vi "Test XML Objects.vi"() -> ()   [LabVIEW 2013]
uses:
  Shifter.lvclass
  Shifters.lvclass
  ACNET Device Limits List.lvclass
  ACNET Device Limits.lvclass
panel:
  out "Device Limits":string
  out "Device Range States":cluster{"name":string, dbl, "Numeric":i8}[](array[cluster]) {"?" format="%_6g"}
  out "Shifter List XML":string
  out "Shifter XML":string
  out "phoneNumbers":string[](array[string])
  out "emails":string[](array[string])
  out "name":string
  in  "XML File Path":path=path "C:/Users/plane/Dropbox/Research/MTA/DAQ VIs/XML Objects/Test Shifter Object.xml"
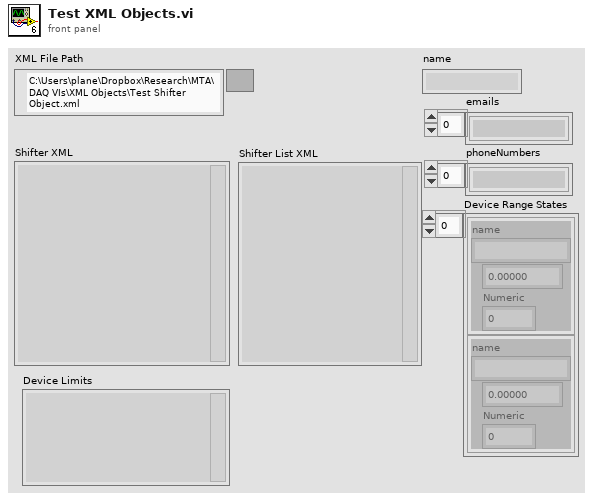
[diagram p1: front panel]
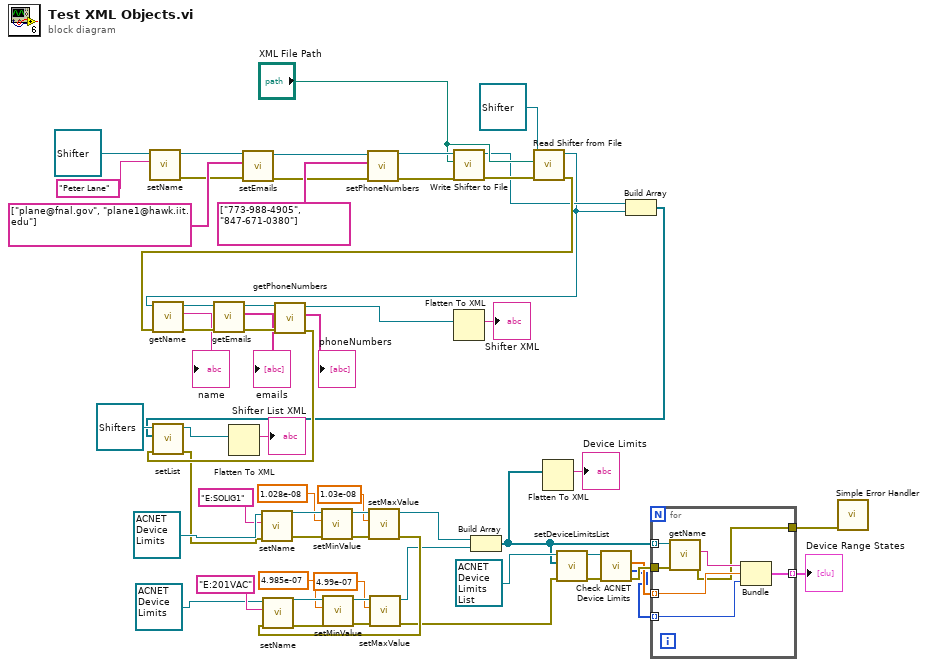
[diagram p0: block diagram]
diagram:
  n1 = call-dynamic "setName.vi"("name"="Peter Lane", "Shifter in"=refnum<class "Shifter.lvclass"> refnum ("Shifter.lvclass")) -> ("error out"=w54:errorcluster, "Shifter out"=w59:refnum<class "Shifter.lvclass">)  [unwired: 8 in]
  n2 = call-dynamic "setEmails.vi"("error in (no error)"=w54, "emails"=string[] ["plane@fnal.gov", "plane1@hawk.iit.edu"], "Shifter in"=w59) -> ("error out"=w53:errorcluster, "Shifter out"=w56:refnum<class "Shifter.lvclass">)  [unwired: 7 in]
  n3 = call-dynamic "setPhoneNumbers.vi"("error in (no error)"=w53, "phoneNumbers"=string[] ["773-988-4905", "847-671-0380"], "Shifter in"=w56) -> ("error out"=w52:errorcluster, "Shifter out"=w55:refnum<class "Shifter.lvclass">)  [unwired: 7 in]
  n4 = call "Write Shifter to File.vi"("error in (no error)"=w52, "XML File Path"="XML File Path", "Shifter in"=w55) -> ("error out"=w51:errorcluster, "Shifter out"=w36:refnum<class "Shifter.lvclass">)  [unwired: 7 in]
  n5 = call "Read Shifter from File.vi"("error in (no error)"=w51, "XML File Path"="XML File Path", "Shifter in"=refnum<class "Shifter.lvclass"> refnum) -> ("error out"=w48:errorcluster, "Shifter out"=w35:refnum<class "Shifter.lvclass">)  [unwired: 7 in]
  n6 = call-dynamic "getName.vi"("error in (no error)"=w48, "Shifter in"=w35) -> ("error out"=w45:errorcluster, "name"=→"name":string, "Shifter out"=w47:refnum<class "Shifter.lvclass">)  [unwired: 7 in]
  n7 = call-dynamic "getEmails.vi"("error in (no error)"=w45, "Shifter in"=w47) -> ("error out"=w44:errorcluster, "emails"=→"emails":string[], "Shifter out"=w46:refnum<class "Shifter.lvclass">)  [unwired: 7 in]
  n8 = call-dynamic "getPhoneNumbers.vi"("error in (no error)"=w44, "Shifter in"=w46) -> ("error out"=w37:errorcluster, "phoneNumbers"=→"phoneNumbers":string[], "Shifter out"=w39:refnum<class "Shifter.lvclass">)  [unwired: 7 in]
  n9 = Flatten To XML(anything=w39) -> (xml string=→"Shifter XML":string)
  n10 = Build Array(w36, w35) -> (w34:refnum<class "Shifter.lvclass">[])
  n11 = call-dynamic "setList.vi"("error in (no error)"=w37, "list"=w34, "Shifters in"=refnum<class "Shifters.lvclass"> refnum) -> ("error out"=w29:errorcluster, "Shifters out"=w33:refnum<class "Shifters.lvclass">)  [unwired: 7 in]
  n12 = Flatten To XML(anything=w33) -> (xml string=→"Shifter List XML":string)
  n13 = call-dynamic "setName.vi"("error in (no error)"=w29, "name"="E:SOLIG1", "ACNET Device Limits in"=refnum<class "ACNET Device Limits.lvclass"> refnum ("ACNET Device Limits.lvclass")) -> ("error out"=w27:errorcluster, "ACNET Device Limits out"=w28:refnum<class "ACNET Device Limits.lvclass">)  [unwired: 7 in]
  n14 = call-dynamic "setMinValue.vi"("error in (no error)"=w27, "minValue"=1.028e-08, "ACNET Device Limits in"=w28) -> ("error out"=w24:errorcluster, "ACNET Device Limits out"=w25:refnum<class "ACNET Device Limits.lvclass">)  [unwired: 7 in]
  n15 = call-dynamic "setMaxValue.vi"("error in (no error)"=w24, "maxValue"=1.03e-08, "ACNET Device Limits in"=w25) -> ("error out"=w17:errorcluster, "ACNET Device Limits out"=w13:refnum<class "ACNET Device Limits.lvclass">)  [unwired: 7 in]
  n16 = call-dynamic "setName.vi"("error in (no error)"=w17, "name"="E:201VAC", "ACNET Device Limits in"=refnum<class "ACNET Device Limits.lvclass"> refnum ("ACNET Device Limits.lvclass")) -> ("error out"=w15:errorcluster, "ACNET Device Limits out"=w21:refnum<class "ACNET Device Limits.lvclass">)  [unwired: 7 in]
  n17 = call-dynamic "setMinValue.vi"("error in (no error)"=w15, "minValue"=4.985e-07, "ACNET Device Limits in"=w21) -> ("error out"=w14:errorcluster, "ACNET Device Limits out"=w19:refnum<class "ACNET Device Limits.lvclass">)  [unwired: 7 in]
  n18 = call-dynamic "setMaxValue.vi"("error in (no error)"=w14, "maxValue"=4.99e-07, "ACNET Device Limits in"=w19) -> ("error out"=w10:errorcluster, "ACNET Device Limits out"=w12:refnum<class "ACNET Device Limits.lvclass">)  [unwired: 7 in]
  n19 = Build Array(w13, w12) -> (w3:refnum<class "ACNET Device Limits.lvclass">[])
  n20 = Flatten To XML(anything=w3) -> (xml string=→"Device Limits":string)
  n21 = call-dynamic "setDeviceLimitsList.vi"("error in (no error)"=w10, "Device Limits List"=w3, "ACNET Device Checker in"=refnum<class "ACNET Device Limits List.lvclass"> refnum ("ACNET Device Checker.lvclass")) -> ("error out"=w9:errorcluster, "ACNET Device Checker out"=w8:refnum<class "ACNET Device Limits List.lvclass">)  [unwired: 7 in]
  n22 = call "Check ACNET Device Limits.vi"("error in (no error)"=w9, "ACNET Device Limits List in"=w8) -> ("error out"=w7:errorcluster, "Range States"=w5:i8[], "Values"=w6:dbl[])  [unwired: 6 in, 1 out]
  n23 = for {
    tunnel: w3 -> [w68] mode=indexing
    tunnel: w7 -> [w67]
    tunnel: w6 -> [w65] mode=indexing
    tunnel: w5 -> [w64] mode=indexing
    tunnel: [w63] -> w4 mode=indexing
    tunnel: [w62] -> w1
    n24 = call-dynamic "getName.vi"("error in (no error)"=w67, "ACNET Device Limits in"=w68) -> ("error out"=w62:errorcluster, "name"=w66:string)  [unwired: 7 in, 1 out]
    n25 = Bundle("name"=w66, w65, "Numeric"=w64) -> (w63:cluster{"name":string, dbl, "Numeric":i8})  [unwired: 1 in]
  }
  "Device Range States" <- w4
  n26 = call <vilib>:"Simple Error Handler.vi"("error in (no error)"=w1) -> ()  [unwired: 4 in, 5 out]
